vi "ExSubCreateFile.vi"(2 "error in (no error)":errorcluster, 3 "File and Display Name":string, 4 "Pulser Handle":u32, 5 "Camera Handle":u32) -> (0 "error out":errorcluster, 1 "Handles Out":T1)   [LabVIEW 2010]
panel:
  # "ExSubCreateFile:\nThis is a SubVI that creates a file,  image \nobjects and returns the handles bundled in a cluster that includes a pulser and camera handle"
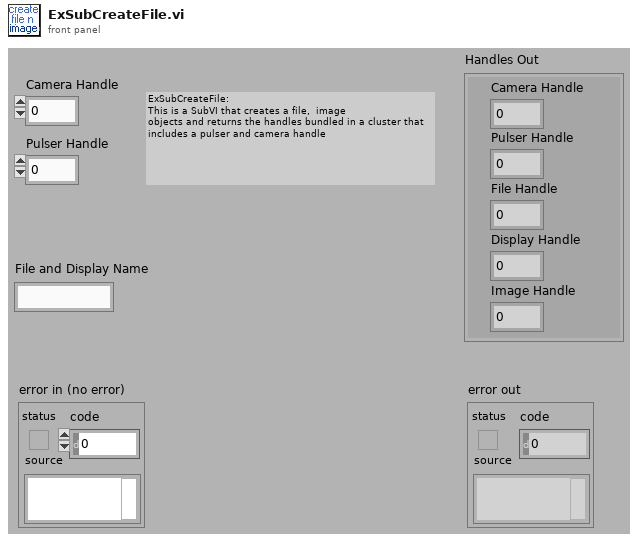
[diagram p1: front panel]
types:
  T1 = cluster{"Camera Handle":u32, "Pulser Handle":u32, "File Handle":u32, "Display Handle":u32, "Image Handle":u32}
  T2 = cluster{"Camera Handle":u32, "Pulser Handle":u32, "File Handle":u32, i32, "Image Handle":u32}
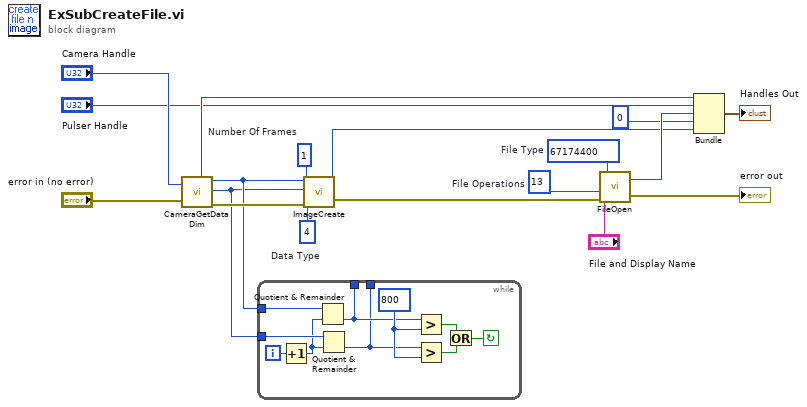
[diagram p0: block diagram]
diagram:
  w7 = u32 1  # Number Of Frames
  w8 = u32 4  # Data Type
  w9 = 13  # File Operations
  w10 = 67174400  # File Type
  n1 = call <userlib>:"CameraGetDataDim.vi"("Camera Handle"="Camera Handle", "error in"="error in (no error)") -> ("Camera Handle"=w14:u32, "Xdim"=w6:u32, "Ydim"=w5:u32, "error out"=w18:errorcluster)
  n2 = while {
    tunnel: w6 -> [w27]
    tunnel: w5 -> [w26]
    tunnel: [w21] -> _
    tunnel: [w20] -> _
    i -> [w25]
    stop <- w22 continue-if-true
    w28 = 800
    n3 = Increment(x=w25) -> (x+1=w19:i32)
    n4 = Quotient & Remainder(x=w27, y=w19) -> (floor(x/y)=w21:u32)  [unwired: 1 out]
    n5 = Quotient & Remainder(x=w26, y=w19) -> (floor(x/y)=w20:u32)  [unwired: 1 out]
    n6 = Greater?(x=w21, y=w28) -> (0:w24:bool)
    n7 = Greater?(x=w20, y=w28) -> (0:w23:bool)
    n8 = Or(x=w24, y=w23) -> (x .or. y?=w22:bool)
  }
  n9 = call <userlib>:"ImageCreate.vi"("X dimension"=w6, "Y dimension"=w5, "Data Type"=w8, "error in"=w18, "Number Of Frames"=w7) -> ("Image Handle"=w11:u32, "error out"=w3:errorcluster)
  n10 = call <userlib>:"FileOpen.vi"("error in"=w3, "File Operations"=w9, "FileName"="File and Display Name", "File Type"=w10) -> ("error out"=→"error out":errorcluster, "File Handle"=w12:u32)
  n11 = Bundle("Camera Handle"=w14, "Pulser Handle"="Pulser Handle", "File Handle"=w12, 0, "Image Handle"=w11) -> (→"Handles Out":T2)  [unwired: 1 in]
